vi "Configure Device.vi"(5 "LNA Gain dB":dbl(knob)=4.5152468054049395 scale=0.0..50.0, 6 "TVA Gain dB":dbl(knob)=4.5152468054049395 scale=0.0..50.0, 7 "Filter Bandwidth":dbl(knob)=5.0 scale=0.0..1.0, 8 "error in (no error)":errorcluster, 9 "Sample frequency":dbl(knob)=8.0 scale=0.0..5.0, 10 "Carrier frequency":dbl(knob)=440.0 scale=0.0..1000.0, 11 "HRF_Device":refnum<class "HRF_Device.lvclass">) -> (0 "error out":errorcluster, 3 "HRF_Device":refnum<class "HRF_Device.lvclass">)   [LabVIEW 2020, in "HRF_Device.lvclass"]
uses:
  HRF_Device.lvclass
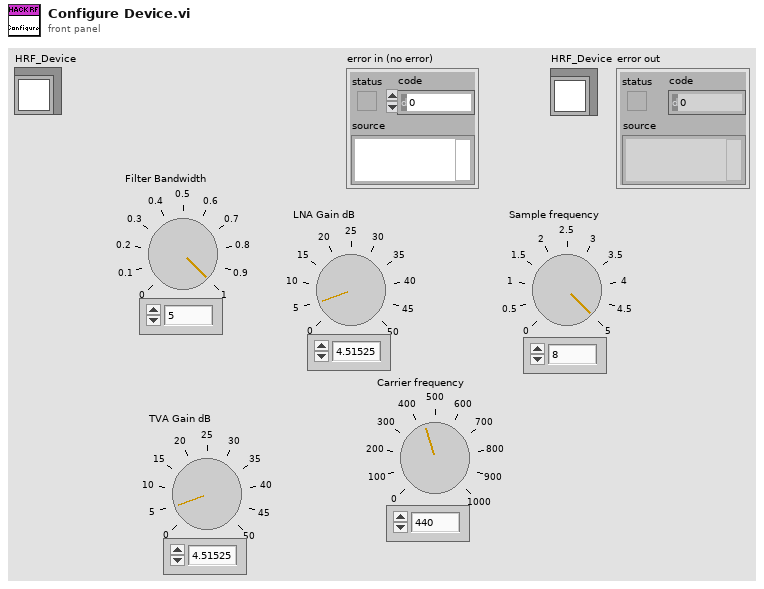
[diagram p1: front panel]
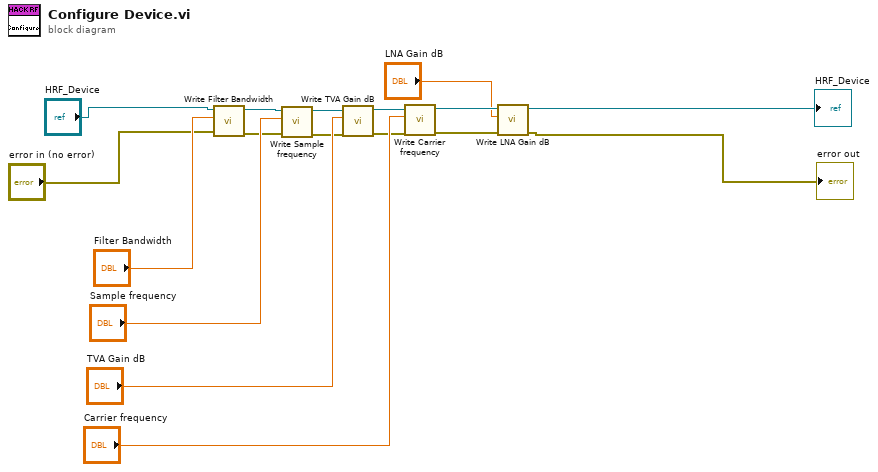
[diagram p0: block diagram]
diagram:
  n1 = call "Write Filter Bandwidth.vi"("error in (no error)"="error in (no error)", "Filter Bandwidth"="Filter Bandwidth", "HRF_Device in"="HRF_Device") -> ("error out"=w10:errorcluster, "HRF_Device out"=w13:refnum<class "HRF_Device.lvclass">)  [unwired: 7 in]
  n2 = call "Write Sample frequency.vi"("error in (no error)"=w10, "Sample frequency"="Sample frequency", "HRF_Device in"=w13) -> ("error out"=w9:errorcluster, "HRF_Device out"=w12:refnum<class "HRF_Device.lvclass">)  [unwired: 7 in]
  n3 = call "Write TVA Gain dB.vi"("error in (no error)"=w9, "TVA Gain dB"="TVA Gain dB", "HRF_Device in"=w12) -> ("error out"=w8:errorcluster, "HRF_Device out"=w11:refnum<class "HRF_Device.lvclass">)  [unwired: 7 in]
  n4 = call "Write Carrier frequency.vi"("error in (no error)"=w8, "Carrier frequency"="Carrier frequency", "HRF_Device in"=w11) -> ("error out"=w5:errorcluster, "HRF_Device out"=w4:refnum<class "HRF_Device.lvclass">)  [unwired: 7 in]
  n5 = call "Write LNA Gain dB.vi"("error in (no error)"=w5, "LNA Gain dB"="LNA Gain dB", "HRF_Device in"=w4) -> ("error out"=→"error out":errorcluster, "HRF_Device out"=→"HRF_Device":refnum<class "HRF_Device.lvclass">)  [unwired: 7 in]
